vi "Main.vi"() -> ()   [LabVIEW 2013]
uses:
  <vilib>/Platform/TimedLoop/XDataNode/timing_clust.ctl
  <vilib>/Platform/TimedLoop/XDataNode/nitl_modes.ctl
  <vilib>/Platform/TimedLoop/XDataNode/wakeup.ctl
  <vilib>/myRIO/Instrument Drivers/Onboard IO/I2C/vis/Smart Open.vi
  <vilib>/myRIO/Instrument Drivers/Onboard IO/I2C/vis/Configure.vi
  <vilib>/myRIO/Instrument Drivers/Onboard IO/I2C/vis/Write.vi
  <vilib>/myRIO/Instrument Drivers/Onboard IO/DIO/vis/Smart Open.vi
  <vilib>/myRIO/Instrument Drivers/Onboard IO/DIO/vis/Read.vi
  <vilib>/myRIO/Instrument Drivers/Onboard IO/I2C/vis/Write Read.vi
  <vilib>/myRIO/Common/Instrument Driver Framework/myRIO v1.0/UART/vis/myRIO v1.0 Close UART.vi
  <vilib>/myRIO/Instrument Drivers/Onboard IO/I2C/vis/Open.vi
  <vilib>/myRIO/Instrument Drivers/Onboard IO/DIO/vis/Open.vi
  <vilib>/myRIO/Common/Instrument Driver Framework/myRIO v1.0/I2C/vis/myRIO v1.1 Open I2C.vi
  <vilib>/myRIO/Common/Instrument Driver Framework/myRIO v1.0/DIO/vis/myRIO v1.1 Open DIO.vi
  <vilib>/myRIO/Common/Instrument Driver Framework/Utilities/vis/Validate Channels.vi
  <vilib>/myRIO/Common/Instrument Driver Framework/myRIO v1.0/I2C/vis/myRIO v1.0 Reserve I2C.vi
  <vilib>/myRIO/Common/Instrument Driver Framework/myRIO v1.0/DIO/vis/myRIO v1.0 Reserve DIO.vi
  <vilib>/myRIO/Common/Instrument Driver Framework/myRIO v1.0/I2C/vis/myRIO v1.0 Build MUX Configuration I2C.vi
  <vilib>/myRIO/Common/Instrument Driver Framework/myRIO v1.0/Resource Manager/vis/myRIO v1.0 Reserve Channel List.vi
  <vilib>/myRIO/Common/Instrument Driver Framework/myRIO v1.0/DIO/vis/myRIO v1.0 Build MUX Configuration DIO.vi
  <vilib>/myRIO/Common/Instrument Driver Framework/myRIO v1.0/Resource Manager/vis/myRIO v1.0 Create Configuration List.vi
  <vilib>/myRIO/Common/Instrument Driver Framework/myRIO v1.0/Resource Manager/vis/myRIO v1.0 Reserve Channel.vi
  <vilib>/myRIO/Common/Instrument Driver Framework/myRIO v1.0/Resource Manager/vis/myRIO v1.0 Unreserve Channel.vi
  <vilib>/myRIO/Common/Instrument Driver Framework/myRIO v1.0/Resource Manager/vis/myRIO v1.0 Build Mutex Name.vi
  <vilib>/myRIO/Common/Instrument Driver Framework/myRIO v1.0/myRIO v1.1 Open.vi
  <vilib>/Utility/VariantDataType/GetNumericInfo.vi
  <vilib>/Utility/error.llb/Error Cluster From Error Code.vi
  <vilib>/myRIO/Common/Instrument Driver Framework/Utilities/vis/IO Manager.vi
  <vilib>/myRIO/Common/Instrument Driver Framework/Utilities/vis/Configuration Manager.vi
  <vilib>/myRIO/Common/Instrument Driver Framework/myRIO v1.0/Resource Manager/vis/myRIO v1.0 Configure IO.vi
  <vilib>/myRIO/Common/Instrument Driver Framework/myRIO v1.0/myRIO v1.0 Close.vi
  <vilib>/myRIO/Common/Instrument Driver Framework/myRIO v1.0/I2C/vis/myRIO v1.0 Configure I2C.vi
  <vilib>/myRIO/Common/Instrument Driver Framework/myRIO v1.0/I2C/vis/myRIO v1.0 Write I2C.vi
  <vilib>/myRIO/Common/Instrument Driver Framework/myRIO v1.0/DIO/vis/myRIO v1.0 Read DIO.vi
  <vilib>/myRIO/Common/Instrument Driver Framework/myRIO v1.0/I2C/vis/myRIO v1.0 Read I2C.vi
  <vilib>/myRIO/Common/Instrument Driver Framework/Utilities/vis/FPGA Ref Manager.vi
  <vilib>/myRIO/Common/Instrument Driver Framework/myRIO v1.0/myRIO v1.0 Reset FPGA.vi
  <vilib>/platform/TimedLoop/XDataNode/XDataNode.xnode
  <vilib>/myRIO/Instrument Drivers/Utilities/Utilities.lvlib
  <vilib>/Platform/TimedLoop/XDataNode/XDNodeRunTimeDep.lvlib
panel:
  out "Magnetic field [LSb]":cluster{i16, i16, i16}(graph) caption="Waveform Chart"
  out "Z":i16
  out "Y":i16
  out "X":i16
  out "DATA":u8[](array[numeric]) format="%02x"
  in  "[ESC]":bool
  # "Compass demo"
  # "DATA_X_H"
  # "DATA_X_L"
  # "DATA_Z_H"
  # "DATA_Z_L"
  # "DATA_Y_H"
  # "DATA_Y_L"
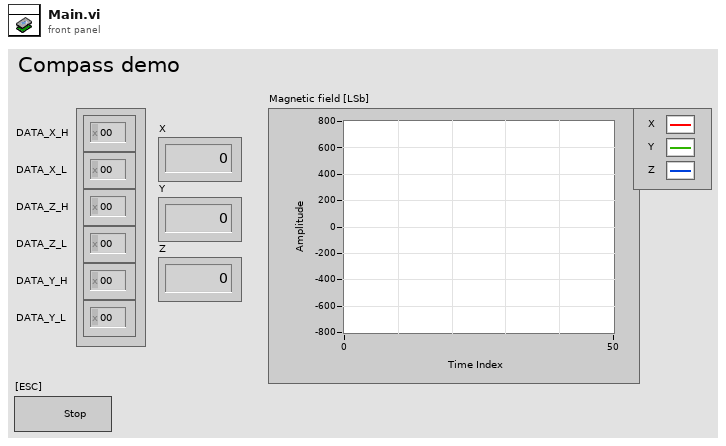
[diagram p1: front panel]
types:
  T1 = typedef "XDNodeRunTimeDep.lvlib/timing_clust.ctl" = cluster{"Expected End [f-1]":u64, "Actual End [f-1]":u64, "Finished Late? [f-1]":bool, "Expected End [i-1]":u64, "Actual End [i-1]":u64, "Finished Late? [i-1]":bool, "Expected Start [i]":u64, "Actual Start [i]":u64, "Expected Start [f]":u64, "Actual Start [f]":u64, "Source Name":string, "Structure Name":string, "Period":i64, "Deadline":i64, "Offset":i64, "Start":i64, "Priority":i32, "Timeout":i32, "Mode":T2, "Wakeup Reason":T3, "Error":errorcluster, "Source Type":string, "Secondary Source Type":string, "Global End Time":u64, "Global Start Time":u64, "Frame Duration":u64, "Iteration Duration":u64, "Assigned CPU":i32, "I/O Scan Engine Mode":u32}
  T2 = typedef "XDNodeRunTimeDep.lvlib/nitl_modes.ctl" = enum32{"No Change", "Process missed periods, maintain original phase", "Discard missed periods, maintain original phase", "Process missed periods, ignore original phase", "Discard missed periods, ignore original phase"}
  T3 = typedef "XDNodeRunTimeDep.lvlib/wakeup.ctl" = enum32{"Normal", "Aborted", "Asynchronous wakeup", "Timing source error", "Timed loop error", "Timeout"}
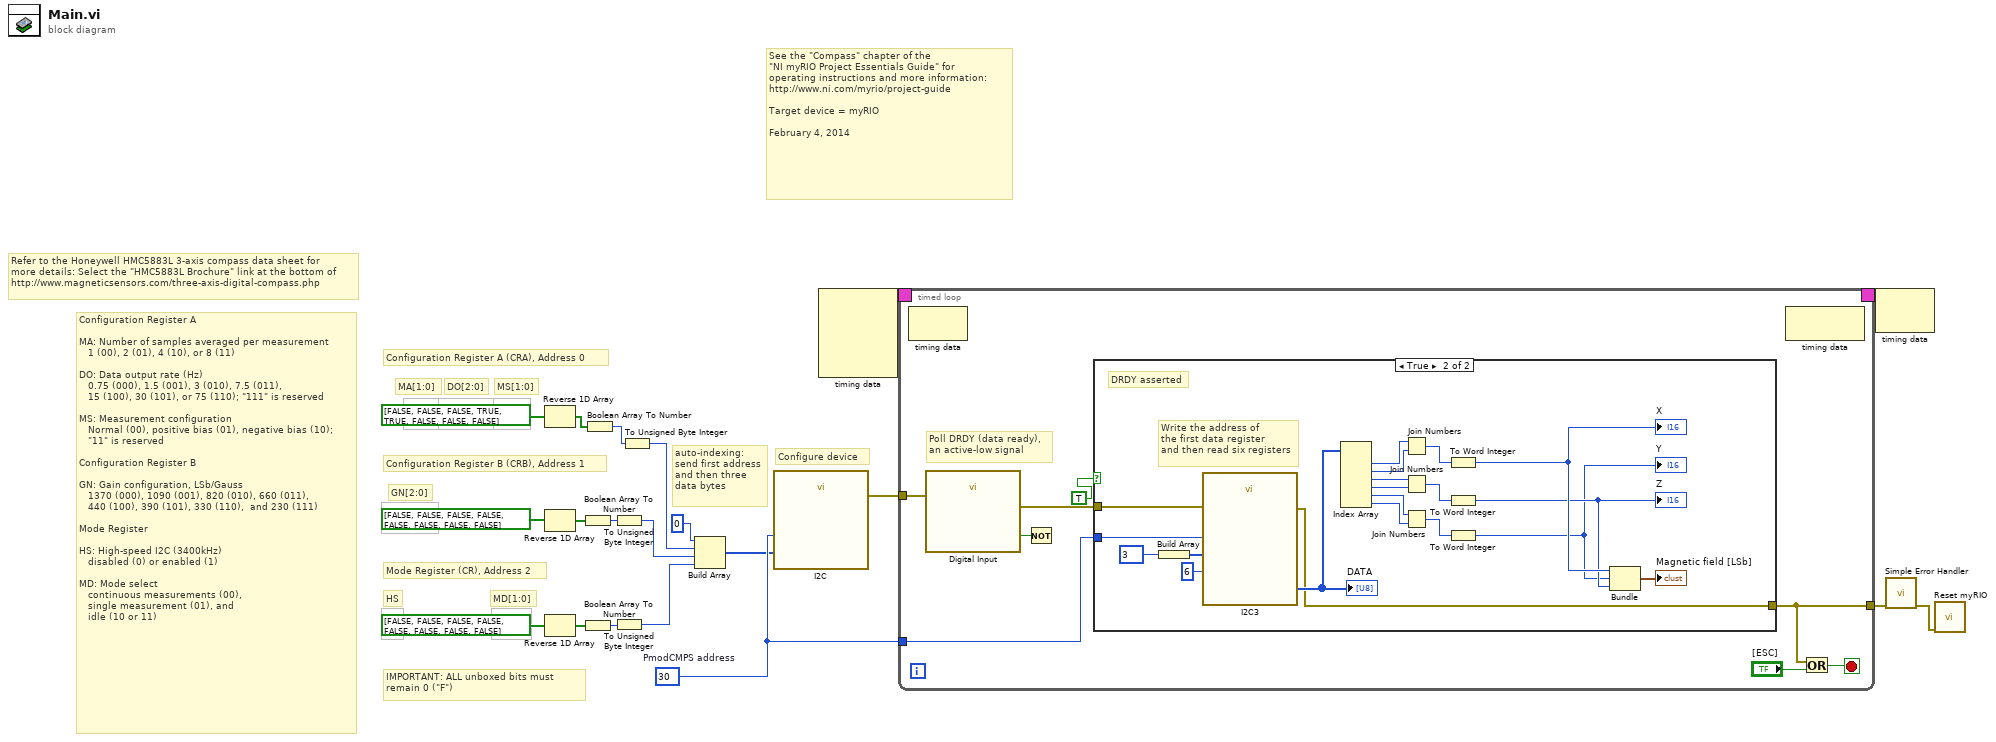
[diagram p0: block diagram]
diagram:
  w17 = u8 30  # PmodCMPS address
  # "See the \"Compass\" chapter of the\n\"NI myRIO Project Essentials Guide\" for\noperating instructions and more information: \nhttp://www.ni.com/myrio/project-guide\n\nTarget device = myRIO\n\nFebruary 4, 2014"
  # "Refer to the Honeywell HMC5883L 3-axis compass data sheet for \nmore details: Select the \"HMC5883L Brochure\" link at the bottom of\nhttp://www.magneticsensors.com/three-axis-digital-compass.php"
  # "auto-indexing:\nsend first address\nand then three\ndata bytes"
  # "Configuration Register A\n\nMA: Number of samples averaged per measurement\n   1 (00), 2 (01), 4 (10), or 8 (11)\n\nDO: Data output rate (Hz)\n   0.75 (000), 1.5 (001), 3 (010), 7.5 (011),\n   15 (100), 30 (101), or 75 (110); \"111\" is reserved\n\nMS: Measurement configuration\n   Normal (00), positive bias (01), negative bias (10);\n   \"11\" is reserved\n\nConfiguration Register B\n\nGN: Gain configuration, LSb/Gauss\n   1370 (000), 1090 (001), 820 (010), 660 (011),\n   440 (100), 390 (101), 330 (110),  and 230 (111)\n\nMode Register\n\nHS: High-speed I2C (3400kHz)\n   disabled (0) or enabled (1)\n\nMD: Mode select\n   continuous measurements (00),\n   single measurement (01), and\n   idle (10 or 11)"
  # "IMPORTANT: ALL unboxed bits must\nremain 0 (\"F\")"
  # "Configure device"
  # "MD[1:0]"
  # "Mode Register (CR), Address 2"
  # "HS"
  # "Configuration Register B (CRB), Address 1"
  # "GN[2:0]"
  # "Configuration Register A (CRA), Address 0"
  # "MS[1:0]"
  # "DO[2:0]"
  # "MA[1:0]"
  n1 = Reverse 1D Array(array=bool[] [FALSE, FALSE, FALSE, TRUE, TRUE, FALSE, FALSE, FALSE]) -> (reversed array=w12:bool[])
  n2 = Reverse 1D Array(array=bool[] [FALSE, FALSE, FALSE, FALSE, FALSE, FALSE, FALSE, FALSE]) -> (reversed array=w11:bool[])
  n3 = Reverse 1D Array(array=bool[] [FALSE, FALSE, FALSE, FALSE, FALSE, FALSE, FALSE, FALSE]) -> (reversed array=w9:bool[])
  n4 = Boolean Array To Number(Boolean array=w11) -> (number=w5:u32)
  n5 = Boolean Array To Number(Boolean array=w9) -> (number=w4:u32)
  n6 = Boolean Array To Number(Boolean array=w12) -> (number=w6:u32)
  n7 = To Unsigned Byte Integer(number=w5) -> (unsigned 8bit integer=w2:u8)
  n8 = To Unsigned Byte Integer(number=w4) -> (unsigned 8bit integer=w1:u8)
  n9 = To Unsigned Byte Integer(number=w6) -> (unsigned 8bit integer=w3:u8)
  n10 = Build Array "Build Array"(u8 0 ("address"), w3, w2, w1) -> (w16:u8[])
  n11 = call "I2C"("Slave Address (7-bit)"=w17, "Bytes to Write"=w16) -> ("error out"=w18:errorcluster)  [unwired: 25 in]
  n12 = node-c288() -> (w15:T1)  [unwired: 4 in]
  n13 = timed-loop {
    tunnel: [w22] -> w19
    tunnel: w18 -> [w25]
    tunnel: w17 -> [w26]
    timing: w15 -> [_]
    timing-out: [_] -> w14
    stop <- w28 stop-if-true
    # "Poll DRDY (data ready),\nan active-low signal"
    n14 = node-c288() -> ()  [unwired: 1 in, 1 out]
    n15 = call "Digital Input"("error in (no error)"=w25) -> ("A/DIO3 (Pin 17)"=w24:bool, "error out"=w23:errorcluster)  [unwired: 25 in]
    n16 = Not(x=w24) -> ()  [unwired: 1 out]
    n17 = case shown="True" TRUE (".not. x?") {
      tunnel: w26 -> [_ w51]
      tunnel: w23 -> [w31 w40]
      tunnel: [w31 w36] -> w22
      frame False {
        # "DRDY deasserted"
      }
      frame True {
        # "DRDY asserted"
        # "Write the address of\nthe first data register\nand then read six registers"
        n18 = Build Array(u8 3) -> (w37:u8[])
        n19 = call "I2C3"("Slave Address (7-bit)"=w51, "Bytes to Write"=w37, "Byte Count"=u32 6, "error in (no error)"=w40) -> ("Bytes Read"=w41:u8[], "error out"=w36:errorcluster)  [unwired: 22 in]
        "DATA" <- w41
        n20 = Index Array "Index Array"(array=w41) -> (element #1=w50:u8, element #2=w49:u8, element #3=w47:u8, element #4=w46:u8, element #5=w45:u8, element #6=w44:u8)  [unwired: 6 in]
        n21 = Join Numbers(hi=w50, lo=w49) -> ((hi.lo)=w48:u16)
        n22 = Join Numbers(hi=w47, lo=w46) -> ((hi.lo)=w43:u16)
        n23 = Join Numbers(hi=w45, lo=w44) -> ((hi.lo)=w42:u16)
        n24 = To Word Integer(number=w48) -> (16bit integer=w34:i16)
        "X" <- w34
        n25 = To Word Integer(number=w43) -> (16bit integer=w33:i16)
        "Z" <- w33
        n26 = To Word Integer(number=w42) -> (16bit integer=w32:i16)
        "Y" <- w32
        n27 = Bundle(w34, w32, w33) -> (→"Magnetic field [LSb]":cluster{i16, i16, i16})  [unwired: 1 in]
      }
    }
    n28 = node-c288() -> ()  [unwired: 1 in, 1 out]
    n29 = Or(x=w22, y="[ESC]") -> (x .or. y?=w28:bool)
  }
  n30 = node-c288(w14) -> ()  [unwired: 1 out]
  n31 = call <vilib>:"Simple Error Handler.vi"("error in (no error)"=w19) -> ("error out"=w20:errorcluster)  [unwired: 4 in, 4 out]
  n32 = call <vilib>:"Reset myRIO.vi"("error in (no error)"=w20) -> ()  [unwired: 10 in, 1 out]
